vi "Read Online_SNR_Frequency.vi"(8 "error in (no error)":errorcluster, 11 "DROPBEAR_Model_Updating in":refnum<class "DROPBEAR_Model_Updating.lvclass">) -> (0 "error out":errorcluster, 2 "Online_SNR.lvclass":refnum<class "Online_SNR.lvclass">, 3 "DROPBEAR_Model_Updating out":refnum<class "DROPBEAR_Model_Updating.lvclass">)   [LabVIEW 2021, in "DROPBEAR_Model_Updating.lvclass"]
uses:
  DROPBEAR_Model_Updating.lvclass
  Online_SNR/Online_SNR.lvclass
  DROPBEAR_Model_Updating.lvclass/DROPBEAR_Model_Updating.ctl
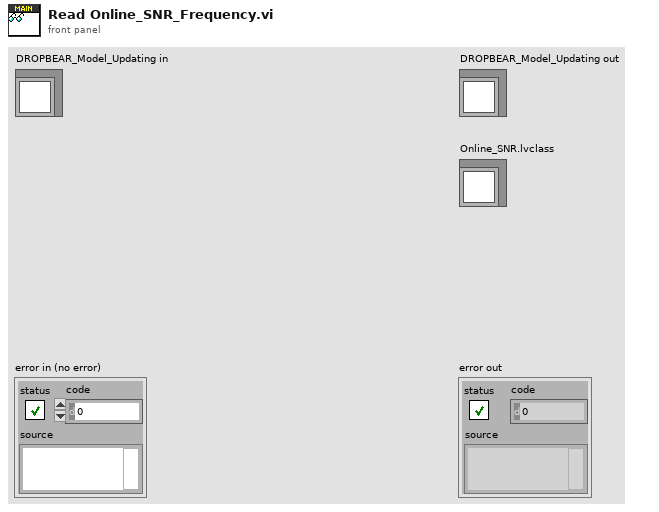
[diagram p1: front panel]
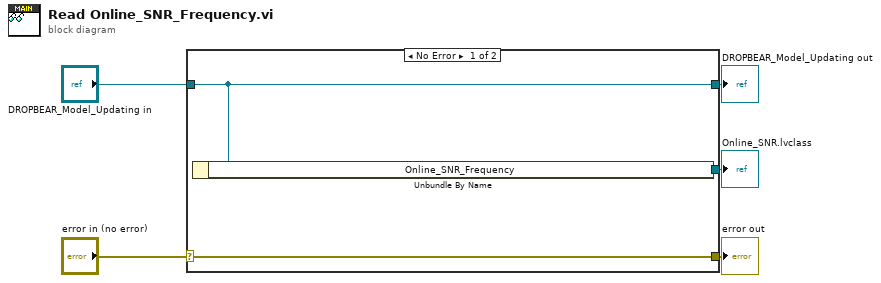
[diagram p0: block diagram]
diagram:
  n1 = case shown="No Error" "error in (no error)" {
    selector: "error in (no error)" -> [w8 w9]
    tunnel: [w8 w9] -> w4
    tunnel: [w7 w10] -> w2
    tunnel: "DROPBEAR_Model_Updating in" -> [w7 w10]
    tunnel: [w6 _] -> w1
    frame No Error {
      n2 = Unbundle By Name(w7) -> ("Online_SNR_Frequency"=w6:refnum<class "Online_SNR.lvclass">)
    }
    frame Error {
    }
  }
  "error out" <- w4
  "DROPBEAR_Model_Updating out" <- w2
  "Online_SNR.lvclass" <- w1
